vi "Acquire DI.vi"(8 "error in (no error)":errorcluster, 11 "PXI 6515 in":refnum<class "PXI 6515.lvclass">) -> (0 "error out":errorcluster, 2 "Acq DI":bool[](array[boolean]), 3 "PXI 6515 out":refnum<class "PXI 6515.lvclass">)   [LabVIEW 2021, in "DAQ IO.lvlib" / "PXI 6515.lvclass"]
uses:
  PXI 6515.lvclass
  <vilib>/DAQmx/read.llb/DAQmx Read (Digital 1D Bool NChan 1Samp 1Line).vi
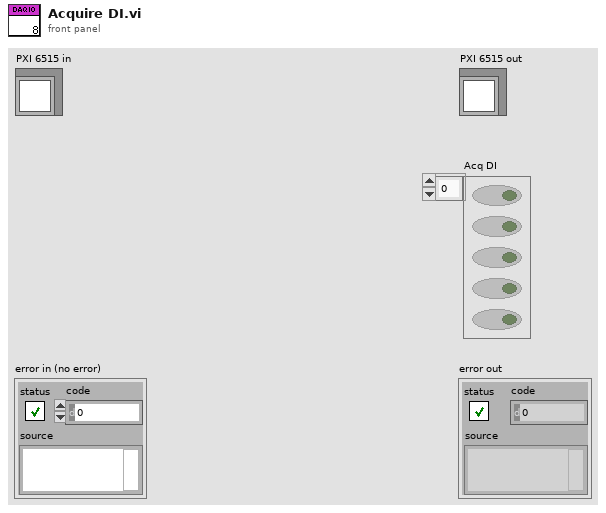
[diagram p1: front panel]
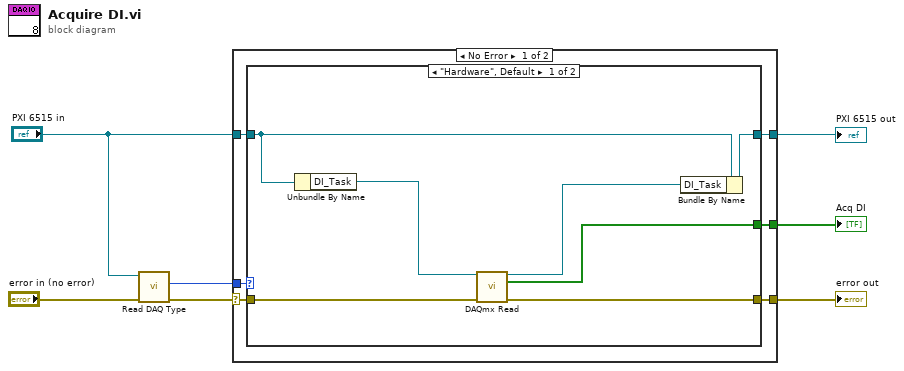
[diagram p0: block diagram]
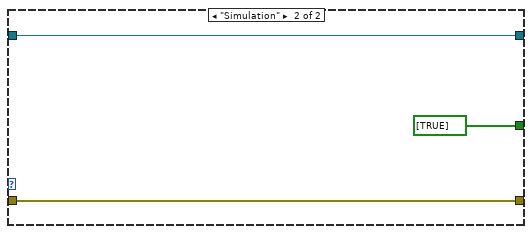
[diagram p2: hidden frame]
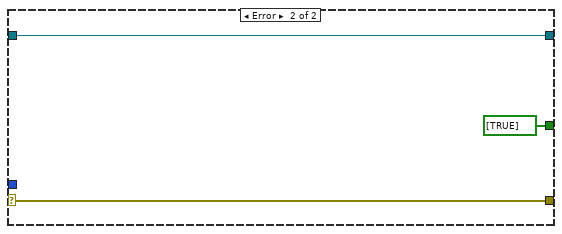
[diagram p3: hidden frame]
diagram:
  n1 = call-dynamic "Read DAQ Type.vi"("error in (no error)"="error in (no error)", "PXI 6515 in"="PXI 6515 in") -> ("error out"=w6:errorcluster, "DAQ Type"=w5:enum16{"Hardware", "Simulation"})  [unwired: 7 in, 1 out]
  n2 = case shown="No Error" w6 {
    selector: w6 -> [w11 w24]
    tunnel: w5 -> [w13 _]
    tunnel: "PXI 6515 in" -> [w12 w26]
    tunnel: [w10 w26] -> w3
    tunnel: [w9 w24] -> w2
    tunnel: [w8 bool[] [TRUE] ("data")] -> w1
    frame No Error {
      n3 = case shown="\"Hardware\", Default" w13 {
        tunnel: w12 -> [w18 w22]
        tunnel: w11 -> [w19 w21]
        tunnel: [w17 w22] -> w10
        tunnel: [w16 w21] -> w9
        tunnel: [w15 bool[] [TRUE] ("data")] -> w8
        frame "Hardware", Default {
          n4 = Unbundle By Name(w18) -> ("DI_Task"=w20:refnum<k21>)
          n5 = call-poly <vilib>:"DAQmx Read.vi"("task/channels in"=w20, "error in"=w19) -> ("task out"=w14:refnum<k21>, "data"=w15:bool[], "error out"=w16:errorcluster)  [unwired: 11 in]
          n6 = Bundle By Name(cluster=w18, "DI_Task"=w14) -> (w17:refnum<class "PXI 6515.lvclass">)
        }
        frame "Simulation" {
        }
      }
    }
    frame Error {
    }
  }
  "error out" <- w2
  "PXI 6515 out" <- w3
  "Acq DI" <- w1
